vi "DSF.Engine.Memory.BufferPool.Set Buffers.vi"(8 "error in (no error)":errorcluster, 10 "Buffers":refnum<class "DSF.Engine.Memory.Buffer.lvclass">[](array[class]), 11 "BufferPool in":refnum<class "DSF.Engine.Memory.BufferPool.lvclass">) -> (0 "error out":errorcluster, 3 "BufferPool out":refnum<class "DSF.Engine.Memory.BufferPool.lvclass">)   [LabVIEW 2016, in "DSF.Engine.lvlib" / "DSF.Engine.Memory.BufferPool.lvclass"]
uses:
  BufferPool/DSF.Engine.Memory.BufferPool.lvclass
  Buffer/DSF.Engine.Memory.Buffer.lvclass
  BufferPool/DSF.Engine.Memory.BufferPool.lvclass/DSF.Engine.Memory.BufferPool.ctl
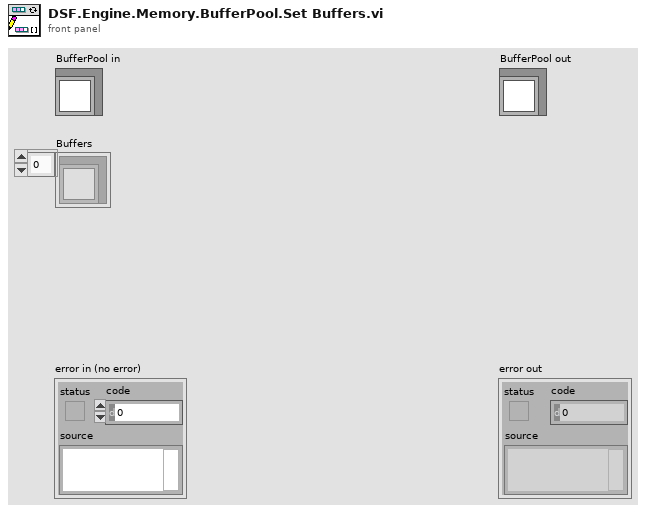
[diagram p1: front panel]
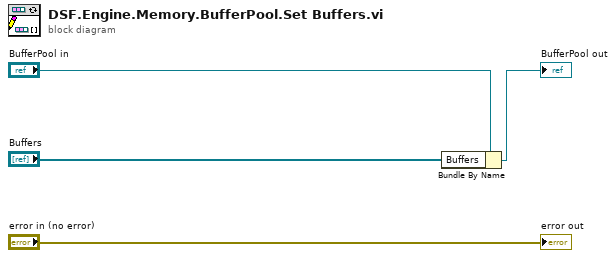
[diagram p0: block diagram]
diagram:
  n1 = Bundle By Name(cluster="BufferPool in", "Buffers"="Buffers") -> (→"BufferPool out":refnum<class "DSF.Engine.Memory.BufferPool.lvclass">)
  "error out" <- "error in (no error)"
